vi "PostProcess.vi"(8 "error in (no error)":errorcluster, 10 "Variant in":variant, 11 "ONNX Class in":refnum<class "ONNX Class.lvclass">) -> (0 "error out":errorcluster, 2 "Variant out":variant, 3 "ONNX Class out":refnum<class "ONNX Class.lvclass">)   [LabVIEW 2017, in "ONNX Class Library.lvlib" / "ONNX Class.lvclass"]
uses:
  ONNX Class.lvclass
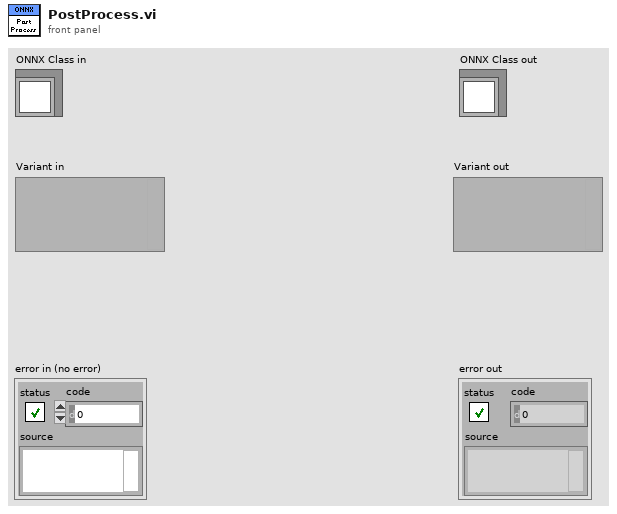
[diagram p1: front panel]
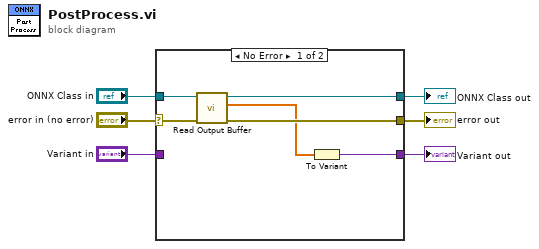
[diagram p0: block diagram]
diagram:
  n1 = case shown="No Error" "error in (no error)" {
    selector: "error in (no error)" -> [w10 w15]
    tunnel: [w9 w15] -> w5
    tunnel: [w11 w14] -> w3
    tunnel: "ONNX Class in" -> [w12 w14]
    tunnel: "Variant in" -> [_ w13]
    tunnel: [w7 w13] -> w1
    frame No Error {
      n2 = call-dynamic "Read Output Buffer.vi"("error in (no error)"=w10, "ONNX Class in"=w12) -> ("error out"=w9:errorcluster, "Output Buffer"=w8:sgl[], "ONNX Class out"=w11:refnum<class "ONNX Class.lvclass">)  [unwired: 7 in]
      n3 = To Variant(anything=w8) -> (Variant=w7:variant)
    }
    frame Error {
    }
  }
  "error out" <- w5
  "ONNX Class out" <- w3
  "Variant out" <- w1
